vi "Howdy.vi"() -> ()   [LabVIEW 2020]
panel:
  in  "message":string="Howdy!"
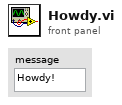
[diagram p1: front panel]
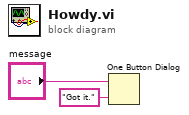
[diagram p0: block diagram]
diagram:
  n1 = One Button Dialog(message="message", button name ("OK")="Got it.") -> ()  [unwired: 1 out]
